vi "util_launch_auto_step.vi"(7 "transition_queue":refnum<queue>, 8 "error in (no error)":errorcluster, 9 "data":variant, 10 "recipe_data":variant, 11 "vi_reference":variant) -> (0 "error out":errorcluster)   [LabVIEW 2015, in "lv-recipe-machine.lvlib"]
uses:
  lv-recipe-machine.lvlib
  _controls/transition.ctl
  _controls/vi_reference_automatic_step.ctl
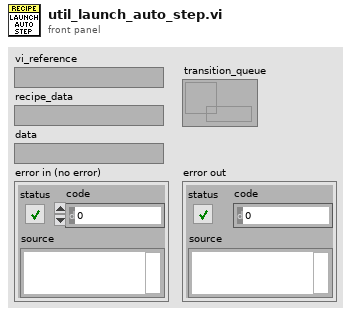
[diagram p1: front panel]
types:
  T1 = typedef "lv-recipe-machine.lvlib/vi_reference_automatic_step.ctl" = refnum<vi>
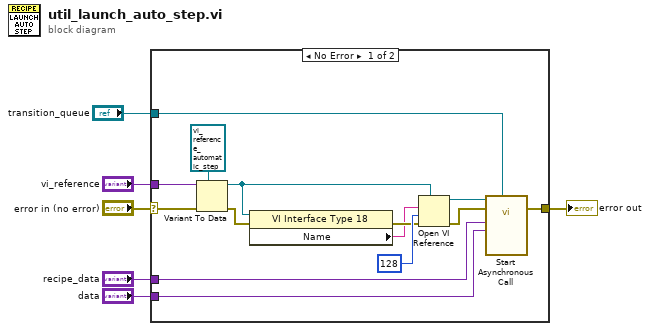
[diagram p0: block diagram]
diagram:
  n1 = case shown="No Error" "error in (no error)" {
    selector: "error in (no error)" -> [w9 w21]
    tunnel: [w19 w21] -> w6
    tunnel: "data" -> [w13 _]
    tunnel: "recipe_data" -> [w12 _]
    tunnel: "vi_reference" -> [w8 _]
    tunnel: "transition_queue" -> [w7 _]
    frame No Error {
      n2 = Variant To Data(error in=w9, type=T1 refnum ("vi_reference_step_action"), Variant=w8) -> (data=w11:T1, error out=w20:errorcluster)
      n3 = property class="VI Interface Type 18"(reference=w11, error in=w20) -> (error out=w16:errorcluster, "Name"=w15:string)  [unwired: 1 out]
      n4 = Open VI Reference(type specifier VI Refnum (for type only)=w11, vi path=w15, options=128, error in (no error)=w16) -> (vi reference=w17:T1, error out=w14:errorcluster)  [unwired: 2 in]
      n5 = call-by-ref "Start Asynchronous Call"(reference=w17, error in=w14, "transition_queue"=w7, "data"=w13, "recipe_data"=w12) -> (error out=w19:errorcluster)  [unwired: 8 in, 2 out]
    }
    frame Error {
    }
  }
  "error out" <- w6
